vi "reverseUnitsConversion.vi"(10 "Units":string, 11 "Time":dbl) -> (3 "Numeric":dbl)   [LabVIEW 2013]
doc: "Converts arbritary floats to a float with one digit in front of the decminal and a a s, ms, mu s or ns string.\nFloats below 1E-11 are rounded to 0."
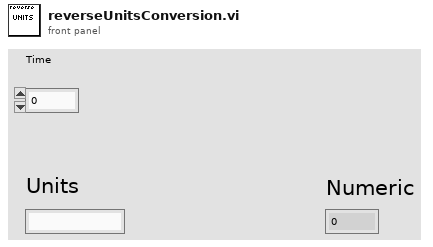
[diagram p1: front panel]
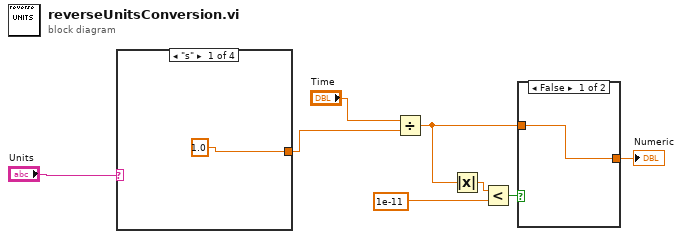
[diagram p0: block diagram]
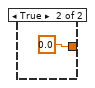
[diagram p2: hidden frame]
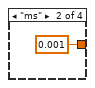
[diagram p3: hidden frame]
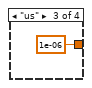
[diagram p4: hidden frame]
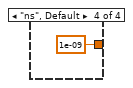
[diagram p5: hidden frame]
diagram:
  n1 = case shown="\"s\"" "Units" {
    tunnel: [1.0 0.001 1e-06 1e-09] -> w6
    frame "s" {
    }
    frame "ms" {
    }
    frame "us" {
    }
    frame "ns", Default {
    }
  }
  n2 = Divide(x="Time", y=w6) -> (x/y=w2:dbl)
  n3 = Absolute Value(x=w2) -> (abs(x)=w1:dbl)
  n4 = Less?(x=w1, y=1e-11) -> (x < y?=w4:bool)
  n5 = case shown="False" w4 {
    tunnel: w2 -> [w13 _]
    tunnel: [w13 0.0] -> w3
    frame False {
    }
    frame True {
    }
  }
  "Numeric" <- w3
